vi "GlobalPlotDataIDTable7.vi"(1 "IO points array size":u32=2048, 2 "IO Data ID in":u32, 3 "Plot channel in":u32, 4 "Function select":string) -> (0 "Plot channel out":u32)   [LabVIEW 2013]
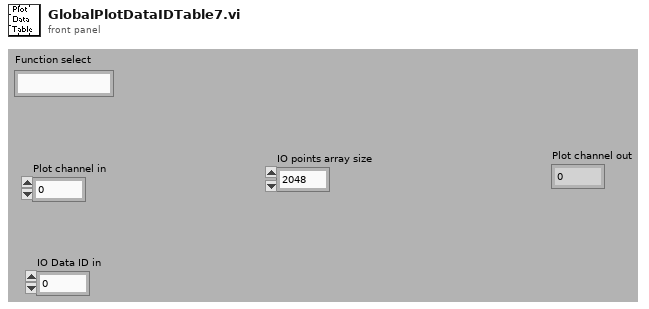
[diagram p1: front panel]
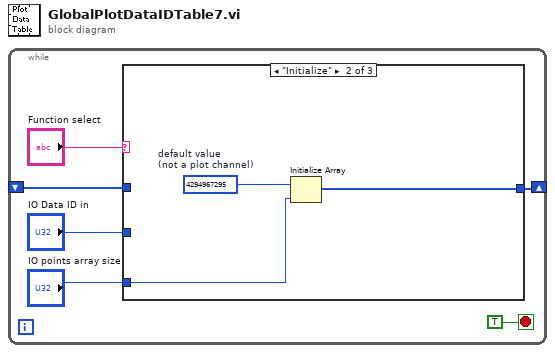
[diagram p0: block diagram]
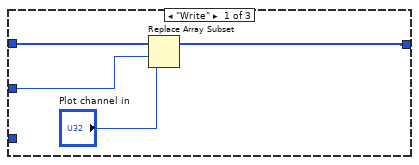
[diagram p2: hidden frame]
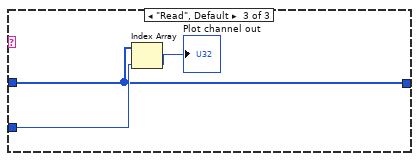
[diagram p3: hidden frame]
diagram:
  n1 = while {
    shift-right: [w4] -> _
    shift-left: _ -> [w3]
    stop <- TRUE stop-if-true
    n2 = case shown="\"Initialize\"" "Function select" {
      tunnel: "IO points array size" -> [_ w13 _]
      tunnel: [w9 w11 w15] -> w4
      tunnel: w3 -> [w10 _ w15]
      tunnel: "IO Data ID in" -> [w8 _ w16]
      frame "Write" {
        n3 = Replace Array Subset(array=w10, new element="Plot channel in", index=w8) -> (w9:u32[])
      }
      frame "Initialize" {
        w12 = u32 4294967295  # default value (not a plot channel)
        n4 = Initialize Array(w12, w13) -> (w11:u32[])
      }
      frame "Read", Default {
        n5 = Index Array(array=w15, index=w16) -> (element=→"Plot channel out":u32)
      }
    }
  }
